vi "WriteCommand.vi"(8 "error in (no error)":errorcluster, 10 "Command":string, 11 "Instrument.Element2 in":refnum<class "Instrument.Element2.lvclass">) -> (0 "error out":errorcluster, 2 "Read Buffer":string, 3 "Instrument.Element2 out":refnum<class "Instrument.Element2.lvclass">)   [LabVIEW 2019, in "Instrument.Element2.lvclass"]
uses:
  Instrument.Element2.lvclass
  Instrument.Element2.lvclass/Instrument.Element2.ctl
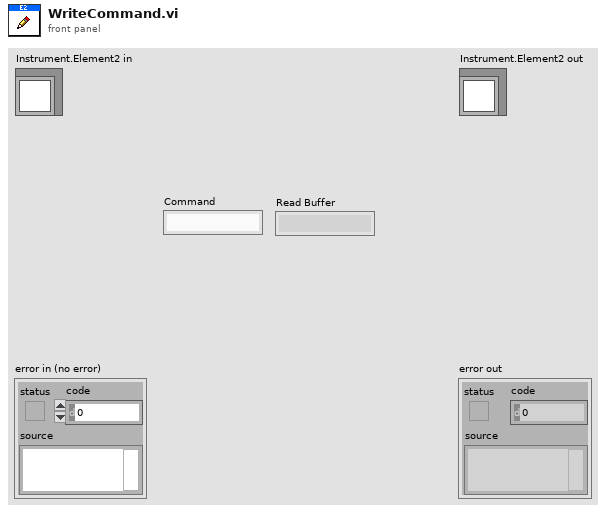
[diagram p1: front panel]
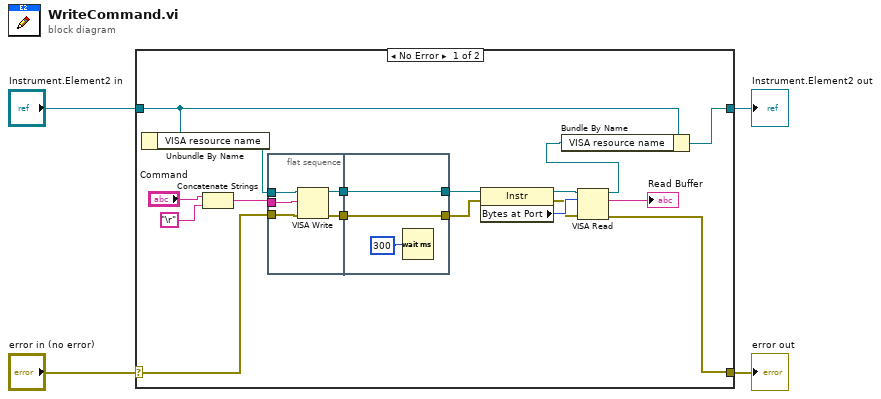
[diagram p0: block diagram]
diagram:
  n1 = case shown="No Error" "error in (no error)" {
    selector: "error in (no error)" -> [w14 w31]
    tunnel: [w13 w31] -> w3
    tunnel: [w10 w30] -> w1
    tunnel: "Instrument.Element2 in" -> [w11 w30]
    frame No Error {
      n2 = Unbundle By Name(w11) -> ("VISA resource name"=w12:refnum<visa-resource-name>)
      n3 = Concatenate Strings("Command", "\r") -> (w5:string)
      n4 = flat-sequence {
        tunnel: [w26] -> w21
        tunnel: [w25] -> w20
        tunnel: w14 -> [w24]
        tunnel: w12 -> [w23]
        tunnel: w5 -> [w22]
        tunnel: [w28] -> w19
        tunnel: w21 -> [w28]
        tunnel: [w27] -> w18
        tunnel: w20 -> [w27]
        frame #0 {
          n5 = VISA Write(VISA resource name=w23, write buffer=w22, error in (no error)=w24) -> (VISA resource name out=w25:refnum<visa-resource-name>, error out=w26:errorcluster)  [unwired: 1 out]
        }
        frame #1 {
          n6 = Wait (ms)(milliseconds to wait=u32 300) -> ()  [unwired: 1 out]
        }
      }
      n7 = property class="Instr"(reference=w18, error in=w19) -> (reference out=w17:refnum<visa-resource-name>, error out=w15:errorcluster, "Bytes at Port"=w16:u32)
      n8 = VISA Read(VISA resource name=w17, byte count=w16, error in (no error)=w15) -> (VISA resource name out=w9:refnum<visa-resource-name>, read buffer=→"Read Buffer":string, error out=w13:errorcluster)  [unwired: 1 out]
      n9 = Bundle By Name(cluster=w11, "VISA resource name"=w9) -> (w10:refnum<class "Instrument.Element2.lvclass">)
    }
    frame Error {
    }
  }
  "error out" <- w3
  "Instrument.Element2 out" <- w1
